vi "Dust_Control_Giraffe_small.vi"(7 "error in":errorcluster) -> (0 "error out":errorcluster)   [LabVIEW 2013]
doc: "This VI specifies the properties of the pulse used for running the dust source. When program is stopped, the voltage is incrementally reduced to zero to avoid quick drops."
uses:
  <vilib>/Utility/miscctls.llb/LVPointTypeDef.ctl
  Global Variables/Action Items.ctl
  <vilib>/Utility/error.llb/DialogType.ctl
  <vilib>/DAQmx/read.llb/DAQmx Read (Analog 1D Wfm NChan NSamp).vi
  <vilib>/Analysis/baseanly.llb/Mean (DBL).vi
  <vilib>/DAQmx/write.llb/DAQmx Write (Analog 1D Wfm NChan NSamp).vi
  <vilib>/DAQmx/read.llb/DAQmx Read (Counter U32 1Chan 1Samp).vi
  <vilib>/addons/database/Connection.llb/Conn Execute.vi
  <vilib>/addons/database/Recordset.llb/Rec Fetch Recordset Data (R).vi
  <vilib>/addons/database/Recordset.llb/Rec Destroy - Connection.vi
  <vilib>/DAQmx/create/channels.llb/DAQmx Create Channel (AI-Voltage-Basic).vi
  <vilib>/DAQmx/configure/timing.llb/DAQmx Timing (Sample Clock).vi
  <vilib>/DAQmx/create/channels.llb/DAQmx Create Channel (AO-Voltage-Basic).vi
  <vilib>/DAQmx/create/channels.llb/DAQmx Create Channel (CI-Count Edges).vi
  <userlib>/_OpenG.lib/comparison/comparison.llb/DBL Changed__ogtk.vi
  <vilib>/measure/mascope.llb/Amplitude and Levels 1 chan.vi
  <vilib>/DAQmx/miscellaneous.llb/DAQmx Fill In Error Info.vi
  Global Variables/throttle.vi
  <userlib>/_OpenG.lib/comparison/comparison.llb/Boolean Changed__ogtk.vi
  Global Variables/throttle from query.vi
  Sub-Polymorphic/post_dust_event_big.vi
  Sub-Polymorphic/post_dust_source_small.vi
  <vilib>/addons/database/_DB Variant To Data/Database Variant To Data.xnode
  <resource>/objmgr/daqmx.rc
  <vilib>/measure/NI_MAPro.lvlib
  <vilib>/Analysis/NI_AALBase.lvlib
  <vilib>/addons/database/NI_Database_API.lvlib
panel:
  out "Freq. Before Throttle":dbl
  out "On/Off":bool
  out "Finished":bool=TRUE
  out "Output waveform":waveform(dbl)={"t0"=timestamp(0 s since 1904-01-01), "dt"=4e-06, "Y"=array[50000 elements]}
  out "Input waveform":waveform(dbl)={"t0"=timestamp(3437998856.0330505 s since 1904-01-01), "dt"=0.00019999999999999998, "Y"=array[1000 elements], "attributes"=variant("NI_ChannelName"=variant(string "Dev5/ai20"), "NI_UnitDescription"=variant(string "Volts"))}
  out "output cluster":T1={"Integer Timestamp"=0, "Needle Voltage"=0.0, "Frequency"=1.0, "Width (ms) : 0.1 "=0.1, "Desired Amplitude (V)"=0.0, "Settings ID"="", "ID#"=0} {"Needle Voltage" min=0.0 max=10.0 step=0.01 format="%.2g"; "Desired Amplitude (V)" min=0.0 max=10.0 step=0.01 format="%5.2f"; "Width (ms) : 0.1" min=0.05 max=5.0 step=0.01 format="%6.2f"; "Frequency" min=1.0 max=100.0 step=0.01 format="%.1f"}
  in  "Tab Control":enum32{"Controls", "Status", "Counter"}(tab)
  in  "Big Accelerator\nSetting?":bool
  out "Actual output width (ms)":dbl caption="Actual Output Width (ms)" format="%.2f"
  out "Actual output Frequency":dbl caption="Actual Output  Frequency (hz)" format="%.2f"
  in  "Width (ms) : 0.1":dbl=0.1 min=0.0 max=5.0 step=0.01 format="%6.2f"
  out "Actual Amplitude (V) 2":dbl=0.0012999050305587314 caption="Actual Amplitude (V)" format="%.2f"
  in  "Desired Amplitude (V)":dbl min=0.0 max=10.0 step=0.01 format="%5.2f"
  out "Actual output Amplitude (V)":dbl caption="Actual Output Amplitude (V)" format="%.2f"
  in  "Frequency":dbl=1.0 caption="Frequency (Hz) : 1" min=0.0 max=30.0 step=0.01 format="%.1f"
  in  "Abort Change":bool
  out "Actual Needle (kV)":dbl=-1.1093266413053247 caption="Actual Einzel (V)" format="%.2f"
  out "Actual Needle Output (V)":dbl caption="Actual Einzel (V)" format="%.2f"
  in  "Needle Voltage":dbl min=0.0 max=10.0 step=0.01 format="%.2g"
  in  "Save Settings?":bool
  out "CONTROLS":waveform(dbl)[](graph)=[{"t0"=timestamp(0 s since 1904-01-01), "dt"=4e-06, "Y"=array[50000 elements]}, {"t0"=timestamp(3437998856.0330505 s since 1904-01-01), "dt"=0.00019999999999999998, "Y"=array[1000 elements], "attributes"=variant("NI_ChannelName"=variant(string "Dev5/ai20"), "NI_UnitDescription"=variant(string "Volts"))}]
  in  "Settings ID":string
  in  "Retrieve Settings":bool
  out "Ratio of particles at\nsecond detector to first":dbl
  out "First detector since\nlast source change:":i64
  out "Average Rate of first":dbl
  out "Average Rate of second":dbl
  in  "# of Cycles ot Average":i32=10
  out "Number of Hours":dbl
  out "Chamber Pressure":dbl format="%#_3g"
  in  "Physical Channels":tag="Dev4/ao0:1" caption="Physical Output Channels"
  in  "Physical Input Channels":tag="Dev6/ai0:2"
  out "Execution Number:":i32=341
  out "Testing":bool
  in  "Counters On/Off":bool=TRUE
  in  "Reset Counters":bool
  in  "Det1":tag="Dev5/ctr0"
  in  "Det2":tag="Dev5/ctr1"
  out "Det2":u32
  out "Det1":u32
  out "error?":bool
  out "Actual Sample Clock Rate":dbl=250000.0 format="%.2f"
  in  "stop":bool
  # "CCLDAS Dust Control Small Accelerator"
  # "Hold Down to\nStop Changes"
  # "Tube Drive (Ao0, Ai4)"
  # "Needle Control (Ao4, Ai0)"
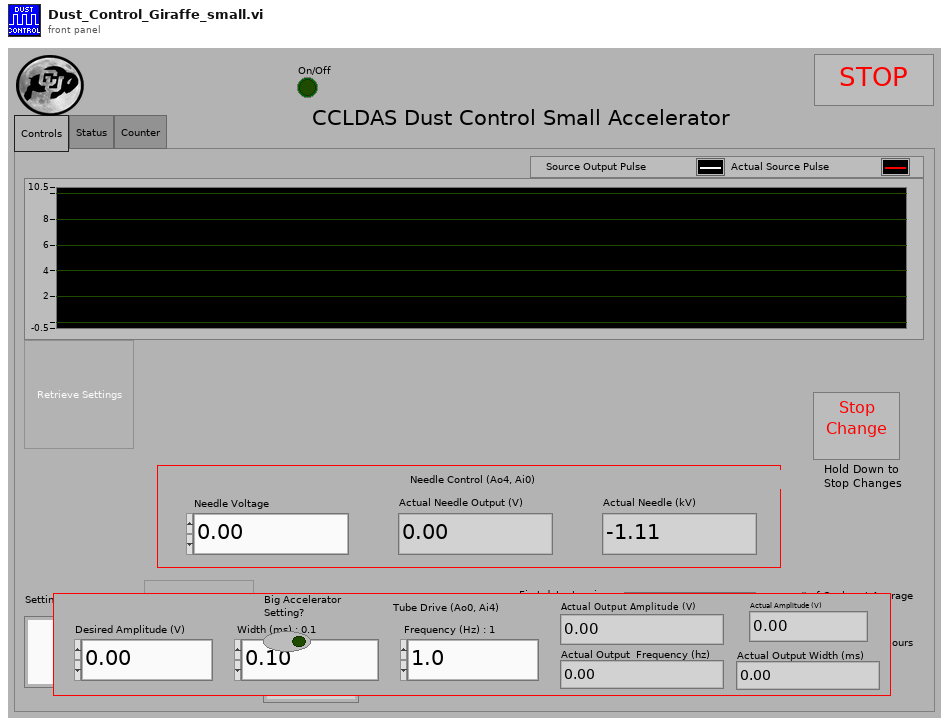
[diagram p1: front panel]
types:
  T1 = cluster{"Integer Timestamp":u64, "Needle Voltage":dbl, "Frequency":dbl, "Width (ms) : 0.1 ":dbl, "Desired Amplitude (V)":dbl, "Settings ID":string, "ID#":i32}
  T2 = typedef "Action Items.ctl" = enum16{"Initialize", "Get", "Set"}
  T3 = typedef "LVPointTypeDef.ctl" = cluster{"Horizontal":i16, "Vertical":i16}
  T4 = typedef "NI_Database_API.lvlib/Conn ObjectReference.ctl" = refnum<k1>
  T5 = typedef "NI_Database_API.lvlib/Rec ObjectReference.ctl" = refnum<k1>
  T6 = enum8{"Enabled", "Disabled", "Disabled and Grayed Out"}
  T7 = typedef "DialogType.ctl" = u16
  T8 = typedef "dust_source_control.ctl" = cluster{"Integer Timestamp":u64, "Einzel Voltage":dbl, "Needle Voltage":dbl, "Frequency":dbl, "Width (ms) : 0.1 ":dbl, "Desired Amplitude (V)":dbl, "X Voltage":dbl, "Y Voltage":dbl, "Settings ID":string, "ID#":i32}
  T9 = cluster{"Integer Time":i64, "Integer Time":i64, "data":i32}
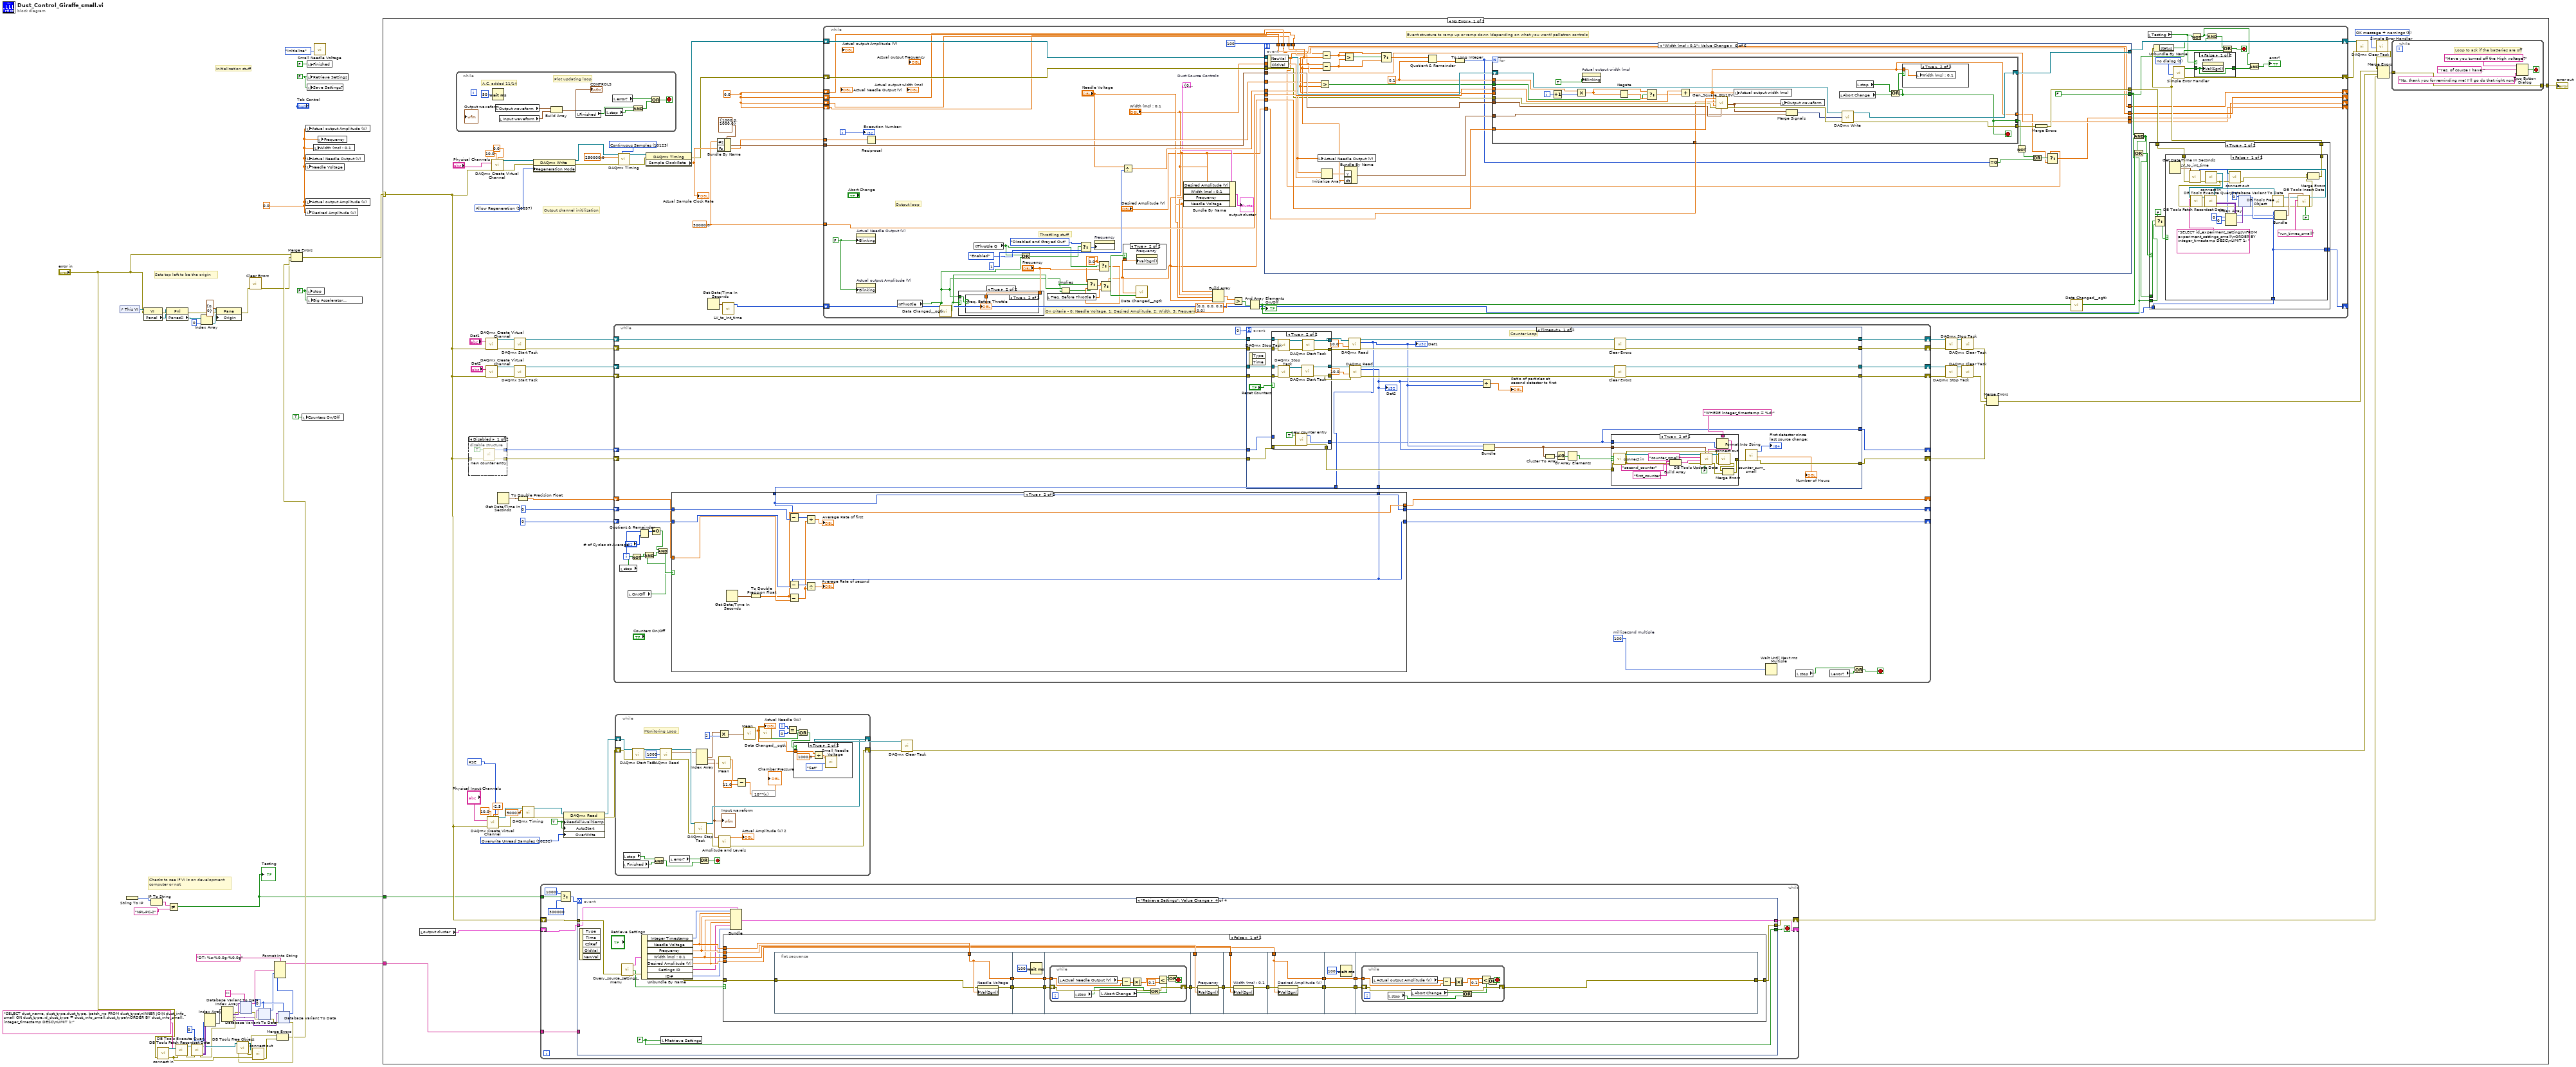
[diagram p0: block diagram]
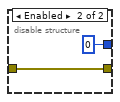
[diagram p2: hidden frame]
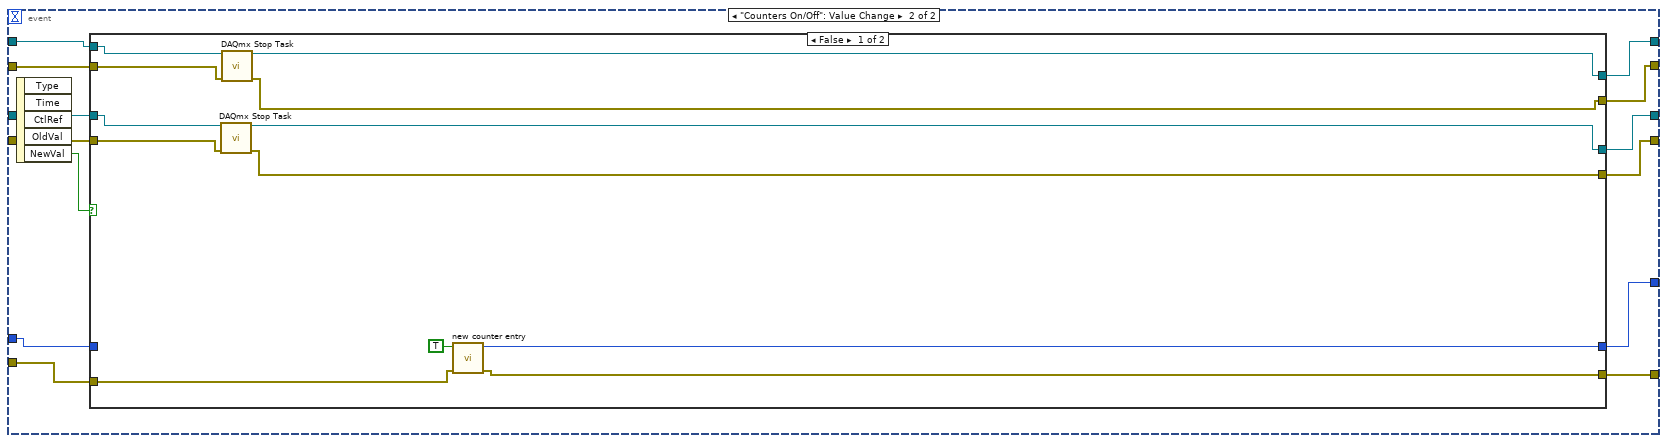
[diagram p5: hidden frame]
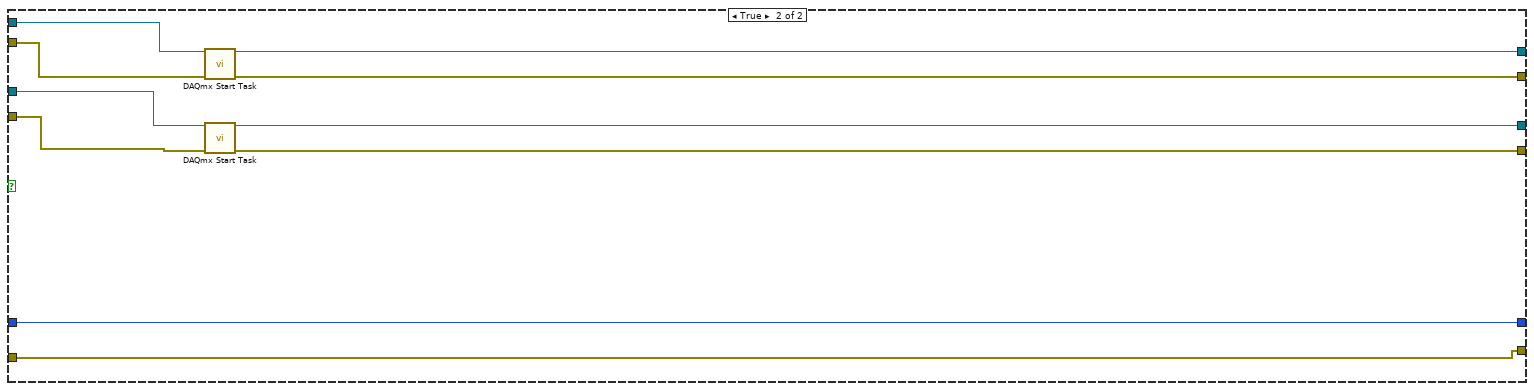
[diagram p6: hidden frame]
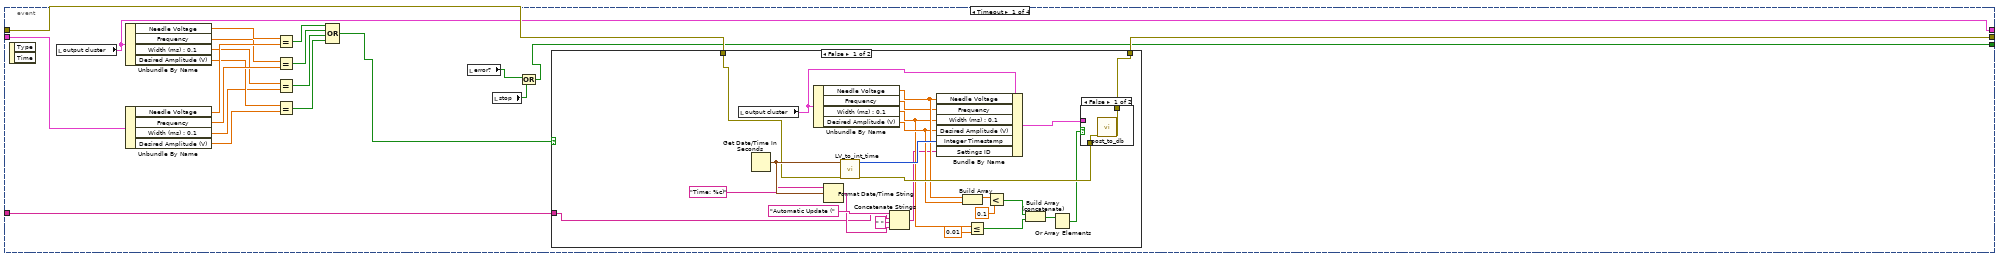
[diagram p9: hidden frame]
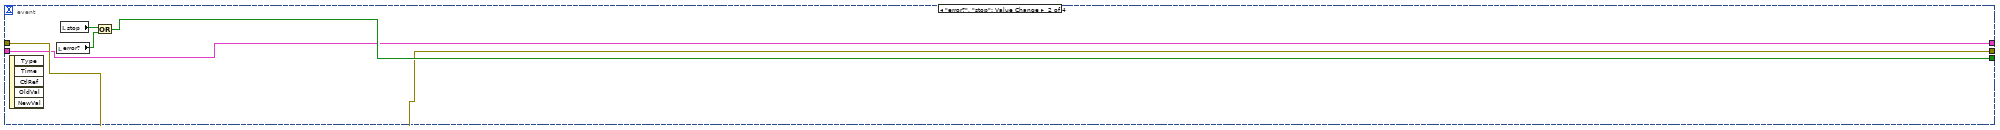
[diagram p12: hidden frame]
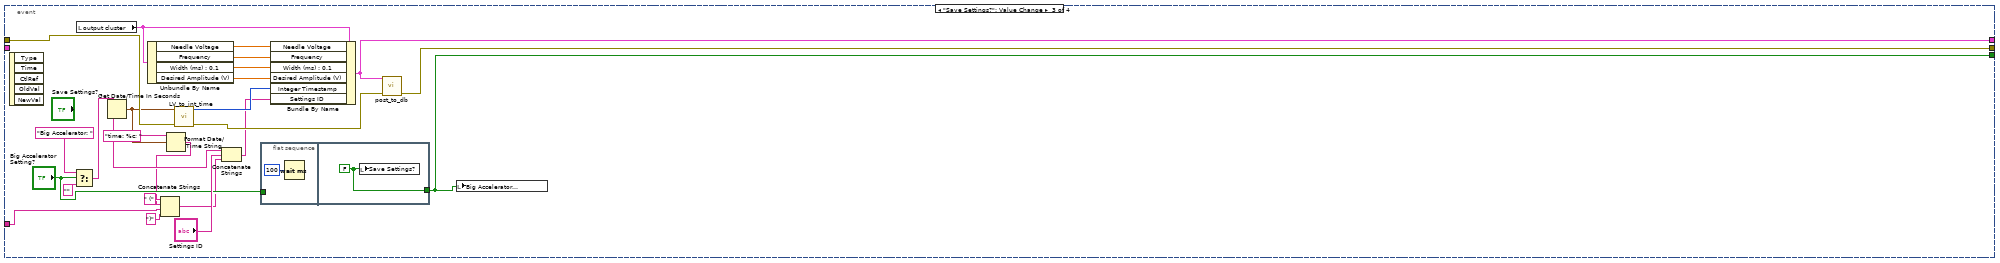
[diagram p13: hidden frame]
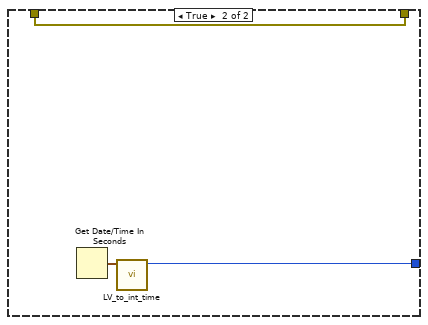
[diagram p19: hidden frame]
diagram:
  w13 = 0
  w48 = FALSE ("Retrieve Settings")
  w46 = 0.0 ("Actual Output (V)")
  w45 = FALSE ("Shutdown")
  # "Checks to see if VI is on development\ncomputer or not"
  # "Sets top left to be the origin"
  # "Initialization stuff"
  n1 = control-ref of="This VI"() -> (w44:refnum<vi>)
  n2 = String To IP() -> (0:w36:u32)  [unwired: 1 in]
  n3 = property class="VI"(reference=w44, error in="error in") -> (error out=w43:errorcluster, "Panel"=w42:refnum<vi>)  [unwired: 1 out]
  n4 = IP To String(2:w36) -> (0:w35:string)  [unwired: 1 in]
  n5 = call "connect in.vi"("error in (no error)"="error in") -> ("error out"=w30:errorcluster, "Database Connection"=w33:T4)  [unwired: 7 in]
  n6 = property class="Pnl"(reference=w42, error in=w43) -> (error out=w41:errorcluster, "Panes[]"=w40:refnum<vi>[])  [unwired: 1 out]
  n7 = Not Equal?(x=w35, y="NPL-PC-2") -> (x != y?=w6:bool)
  "Testing" <- w6
  n8 = call-poly <vilib>:"DB Tools Execute Query.vi"("error in (no error)"=w30, "SQL query"="SELECT dust_name, dust_type.dust_type, batch_no FROM dust_type\nINNER JOIN dust_info_small ON dust_type.id_dust_type = dust_info_small.dust_type\nORDER BY dust_info_small.integer_timestamp DESC\nLIMIT 1;", "connection reference"=w33) -> ("error out"=w32:errorcluster, "recordset reference"=w31:T5)  [unwired: 5 in]
  n9 = call-poly <vilib>:"DB Tools Fetch Recordset Data.vi"("error in (no error)"=w32, "recordset reference"=w31) -> ("error out"=w18:errorcluster, "recordset data"=w28:variant[][], "recordset reference out"=w27:T5)  [unwired: 3 in]
  n10 = Index Array(array=w40, index=0) -> (element=w38:refnum<vi>)
  n11 = Index Array(array=w28, index (row)=0) -> (element=w22:variant[])  [unwired: 1 in]
  n12 = property class="Pane"(reference=w38, error in=w41, "Origin"=T3 {"Horizontal"=0, "Vertical"=0}) -> (error out=w3:errorcluster)  [unwired: 1 out]
  n13 = Index Array(array=w22) -> (element #1=w21:variant, element #2=w16:variant, element #3=w15:variant)  [unwired: 3 in]
  n14 = xnode "Database Variant To Data"("database variant"=w21, "error in (no error)"=w18, "type"="") -> ("data"=w11:string, "error out"=w20:errorcluster)
  n15 = call <vilib>:"Clear Errors.vi"("error in (no error)"=w3) -> ("error out"=w4:errorcluster)  [unwired: 6 in]
  n16 = xnode "Database Variant To Data"("database variant"=w16, "error in (no error)"=w20, "type"=w13) -> ("data"=w10:i32, "error out"=w19:errorcluster)
  n17 = xnode "Database Variant To Data"("database variant"=w15, "error in (no error)"=w19, "type"=w13) -> ("data"=w9:i32, "error out"=w17:errorcluster)
  n18 = call-poly <vilib>:"DB Tools Free Object.vi"("error in (no error)"=w17, "recordset reference"=w27) -> ("error out"=w26:errorcluster, "connection reference"=w23:T4)  [unwired: 8 in]
  n19 = call "connect out.vi"("error in (no error)"=w30, "connection reference"=w23) -> ("error out"=w25:errorcluster)  [unwired: 9 in]
  n20 = Format Into String(format string="DT: %s-%0.0g-%0.0g", w11, w10, w9) -> (resulting string=w7:string)  [unwired: 2 in, 1 out]
  n21 = Merge Errors(w26, w25) -> (w8:errorcluster)
  n22 = Merge Errors("error in", w4, w8) -> (w5:errorcluster)
  n23 = local write "Counters On/Off"(TRUE ("Counters On/Off")) -> ()
  n24 = local write "Actual output Amplitude (V)"(w46) -> ()
  n25 = local write "Actual Needle Output (V)"(w46) -> ()
  n26 = local write "Needle Voltage"(w46) -> ()
  n27 = local write "Actual output Amplitude (V)"(w46) -> ()
  n28 = local write "Desired Amplitude (V)"(w46) -> ()
  n29 = local write "Finished"(FALSE ("Finished")) -> ()
  n30 = local write "Retrieve Settings"(w48) -> ()
  n31 = local write "Save Settings?"(w48) -> ()
  n32 = local write "stop"(w45) -> ()
  n33 = local write "Big Accelerator\nSetting?"(w45) -> ()
  n34 = local write "Width (ms) : 0.1"(w46) -> ()
  n35 = call "Small Needle Voltage.vi"("Action"=Action_Items."Initialize") -> ()  [unwired: 10 in, 1 out]
  n36 = local write "Frequency"(w46) -> ()
  n37 = case shown="No Error" w5 {
    selector: w5 -> [w63 w996]
    tunnel: [w105 w996] -> w50
    tunnel: w7 -> [w53 _]
    tunnel: w6 -> [w52 _]
    frame No Error {
      w51 = 10083 items=["default"=-1, "RSE"=10083, "NRSE"=10078, "Differential"=10106, "Pseudodifferential"=12529] ("input terminal configuration")
      w60 = 0.0 ("Width (ms) : 3.5")
      w73 = 10252 items=["Overwrite Unread Samples"=10252, "Do Not Overwrite Unread Samples"=10159] ("OverWrite")
      w74 = TRUE ("ReadAllAvailSamp")
      w56 = 50000.0 ("Size (Samples)")
      w118 = 10097 items=["Allow Regeneration"=10097, "Do Not Allow Regeneration"=10158] ("RegenMode")
      w123 = T7 3 items=["no dialog", "OK message", "continue or stop message", "OK message + warnings", "continue/stop + warnings"] ("type of dialog (OK msg:1)")
      w127 = 10123 items=["Finite Samples"=10178, "Continuous Samples"=10123] ("sample mode")
      # "Output channel initilization"
      n38 = local read "output cluster"() -> (w55:T1)
      n39 = while {
        stop <- w302 stop-if-true
        # "Plot updating loop"
        # "A.C. added 11/14"
        n40 = Wait (ms)(milliseconds to wait=u32 50) -> ()  [unwired: 1 out]
        n41 = local read "Output waveform"() -> (w299:waveform(dbl))
        n42 = local read "Input waveform"() -> (w300:waveform(dbl))
        n43 = Build Array(w299, w300) -> (→"CONTROLS":waveform(dbl)[])
        n44 = local read "Finished"() -> (w297:bool)
        n45 = local read "stop"() -> (w298:bool)
        n46 = local read "error?"() -> (w301:bool)
        n47 = And(x=w297, y=w298) -> (x .and. y?=w296:bool)
        n48 = Or(x=w301, y=w296) -> (x .or. y?=w302:bool)
      }
      n49 = disable-structure shown="Disabled" {
        disable-tunnel: [w131 w133] -> w82
        disable-tunnel: [w130 i64 0 ("Integer Time")] -> w81
        disable-tunnel: w63 -> [w129 w133]
        frame Disabled {
          n50 = call "new counter entry.vi"("error in"=w129, "Small?"=TRUE) -> ("error out"=w131:errorcluster, "Integer Time"=w130:i64)  [unwired: 8 in]
        }
        frame Enabled {
        }
      }
      n51 = call-poly <vilib>:"DAQmx Create Virtual Channel.vi"("counter"="Det1", "error in"=w63) -> ("task out"=w90:refnum<k21>, "error out"=w87:errorcluster)  [unwired: 12 in]
      n52 = call-poly <vilib>:"DAQmx Create Virtual Channel.vi"("counter"="Det2", "error in"=w63) -> ("task out"=w89:refnum<k21>, "error out"=w88:errorcluster)  [unwired: 12 in]
      n53 = call-poly <vilib>:"DAQmx Create Virtual Channel.vi"("maximum value"=10.0 ("Maximum Value"), "minimum value"=-2.5 ("Minimum Value"), "input terminal configuration"=w51, "physical channels"="Physical Input Channels", "error in"=w63) -> ("task out"=w67:refnum<k21>, "error out"=w66:errorcluster)  [unwired: 9 in]
      n54 = call-poly <vilib>:"DAQmx Create Virtual Channel.vi"("maximum value"=10.0 ("Maximum Value"), "minimum value"=0.0 ("Minimum Value"), "physical channels"="Physical Channels", "error in"=w63) -> ("task out"=w117:refnum<k21>, "error out"=w116:errorcluster)  [unwired: 10 in]
      n55 = Get Date/Time In Seconds() -> (seconds since 1Jan1904=w80:timestamp)
      n56 = call <vilib>:"DAQmx Start Task.vi"("task/channels in"=w90, "error in"=w87) -> ("task out"=w102:refnum<k21>, "error out"=w99:errorcluster)  [unwired: 12 in]
      n57 = call <vilib>:"DAQmx Start Task.vi"("task/channels in"=w89, "error in"=w88) -> ("task out"=w101:refnum<k21>, "error out"=w100:errorcluster)  [unwired: 12 in]
      n58 = To Double Precision Float(number=w80) -> (double precision float=w79:dbl)
      n59 = call-poly <vilib>:"DAQmx Timing.vi"("task/channels in"=w67, "rate"=5000.0, "error in"=w66) -> ("task out"=w72:refnum<k21>, "error out"=w71:errorcluster)  [unwired: 11 in]
      n60 = property class="DAQmx Write"(reference=w117, error in=w116, "Regeneration Mode"=w118) -> (reference out=w115:refnum<k21>, error out=w114:errorcluster)
      n61 = while {
        shift-right: [w348] -> w84
        shift-left: w63 -> [w347]
        shift-right: [w340] -> _
        shift-left: w55 -> [w349]
        tunnel: w52 -> [w343]
        tunnel: w53 -> [w341]
        stop <- w346 stop-if-true
        n62 = Select(t=1000, s=w343, f=300000) -> (s? t:f=w345:i32)
        n63 = event shown="[3] \"Retrieve Settings\": Value Change" {
          selector: _ -> [_ _ _ _]
          dyn-events: _ -> [_ _ _ _]
          timeout: w345 -> [_ _ _ _]
          tunnel: [w350 w399 w404 w430] -> w340
          tunnel: w349 -> [w370 w399 _ w438]
          tunnel: [w355 w400 w427 w444] -> w348
          tunnel: w347 -> [w356 w400 w424 w442]
          tunnel: [w353 w401 w413 w443] -> w346
          tunnel: w341 -> [w357 _ w410 _]
          event Timeout {
            n64 = event-data() -> ()  [unwired: 1 in, 2 out]
            n65 = local read "output cluster"() -> (w350:T1)
            n66 = Unbundle By Name(w350) -> ("Needle Voltage"=w369:dbl, "Frequency"=w367:dbl, "Width (ms) : 0.1"=w365:dbl, "Desired Amplitude (V)"=w363:dbl)
            n67 = Unbundle By Name(w370) -> ("Needle Voltage"=w368:dbl, "Frequency"=w366:dbl, "Width (ms) : 0.1"=w358:dbl, "Desired Amplitude (V)"=w364:dbl)
            n68 = Equal?(x=w369, y=w368) -> (x = y?=w362:bool)
            n69 = Equal?(x=w367, y=w366) -> (x = y?=w361:bool)
            n70 = Equal?(x=w365, y=w358) -> (x = y?=w360:bool)
            n71 = Equal?(x=w363, y=w364) -> (x = y?=w359:bool)
            n72 = Compound Arithmetic op=OR(w362, w361, w360, w359) -> (w354:bool)
            n73 = local read "error?"() -> (w352:bool)
            n74 = local read "stop"() -> (w351:bool)
            n75 = Or(x=w352, y=w351) -> (x .or. y?=w353:bool)
            n76 = case shown="False" w354 {
              tunnel: w357 -> [w371 _]
              tunnel: w356 -> [w376 w398]
              tunnel: [w375 w398] -> w355
              frame False {
                n77 = local read "output cluster"() -> (w380:T1)
                n78 = Get Date/Time In Seconds() -> (seconds since 1Jan1904=w392:timestamp)
                n79 = Unbundle By Name(w380) -> ("Needle Voltage"=w390:dbl, "Frequency"=w386:dbl, "Width (ms) : 0.1"=w385:dbl, "Desired Amplitude (V)"=w389:dbl)
                n80 = Format Date/Time String(time format string (%c)="Time: %c)" ("Settings ID"), seconds (now)=w392) -> (date/time string=w372:string)  [unwired: 1 in]
                n81 = call "LV_to_int_time.vi"("error in (no error)"=w376, "Time Stamp"=w392) -> ("error out"=w393:errorcluster, "Integer Time"=w394:i64)  [unwired: 7 in]
                n82 = Concatenate Strings("Automatic Update (" ("string"), w371, " " ("string"), w372) -> (w378:string)
                n83 = Bundle By Name(cluster=w380, "Needle Voltage"=w390, "Frequency"=w386, "Width (ms) : 0.1"=w385, "Desired Amplitude (V)"=w389, "Integer Timestamp"=w394, "Settings ID"=w378) -> (w381:T1)
                n84 = Build Array(w390, w389) -> (w388:dbl[])
                n85 = Less Or Equal?(x=w385, y=0.01) -> (x <= y?=w379:bool)
                n86 = Less?(x=w388, y=0.1) -> (x < y?=w383:bool[])
                n87 = Build Array (concatenate)(w383, w379) -> (w382:bool[])
                n88 = Or Array Elements(Boolean array=w382) -> (logical OR=w377:bool)
                n89 = case shown="False" w377 {
                  tunnel: w381 -> [_ _]
                  tunnel: [w396 w397] -> w375
                  tunnel: w393 -> [w395 w397]
                  frame False {
                    n90 = call-poly "post_to_db.vi"("error in (no error)"=w395) -> ("error out"=w396:errorcluster)  [unwired: 8 in, 2 out]
                  }
                  frame True {
                  }
                }
              }
              frame True {
              }
            }
          }
          event "error?", "stop": Value Change {
            n91 = event-data() -> ()  [unwired: 1 in, 5 out]
            n92 = local read "error?"() -> (w402:bool)
            n93 = local read "stop"() -> (w403:bool)
            n94 = Or(x=w403, y=w402) -> (x .or. y?=w401:bool)
          }
          event "Save Settings?": Value Change {
            n95 = event-data() -> ()  [unwired: 1 in, 5 out]
            n96 = Select(t="Big Accelerator: ", s="Big Accelerator\nSetting?", f="") -> (s? t:f=w415:string)
            n97 = local read "output cluster"() -> (w405:T1)
            n98 = Get Date/Time In Seconds() -> (seconds since 1Jan1904=w422:timestamp)
            n99 = Unbundle By Name(w405) -> ("Needle Voltage"=w421:dbl, "Frequency"=w420:dbl, "Width (ms) : 0.1"=w419:dbl, "Desired Amplitude (V)"=w418:dbl)
            n100 = Format Date/Time String(time format string (%c)="time: %c; " ("Settings ID"), seconds (now)=w422) -> (date/time string=w408:string)  [unwired: 1 in]
            n101 = Concatenate Strings(" (" ("string"), w408, w410, ")" ("string")) -> (w407:string)
            n102 = call "LV_to_int_time.vi"("error in (no error)"=w424, "Time Stamp"=w422) -> ("error out"=w425:errorcluster, "Integer Time"=w426:i64)  [unwired: 7 in]
            n103 = Concatenate Strings(w415, "Settings ID", w407) -> (w406:string)
            n104 = flat-sequence {
              tunnel: "Big Accelerator\nSetting?" -> [_]
              tunnel: [w429] -> w413
              frame #0 {
                n105 = Wait (ms)(milliseconds to wait=u32 100) -> ()  [unwired: 1 out]
              }
              frame #1 {
                w429 = FALSE
                n106 = local write "Save Settings?"(w429) -> ()
              }
            }
            n107 = Bundle By Name(cluster=w405, "Needle Voltage"=w421, "Frequency"=w420, "Width (ms) : 0.1"=w419, "Desired Amplitude (V)"=w418, "Integer Timestamp"=w426, "Settings ID"=w406) -> (w404:T1)
            n108 = call-poly "post_to_db.vi"("error in (no error)"=w425, "Dust control settings"=w404) -> ("error out"=w427:errorcluster)  [unwired: 9 in]
            n109 = local write "Big Accelerator\nSetting?"(w413) -> ()
          }
          event "Retrieve Settings": Value Change {
            w443 = FALSE
            n110 = event-data() -> ()  [unwired: 1 in, 5 out]
            n111 = call "Query_source_settings_menu.vi"("error in (no error)"=w442) -> ("error out"=w440:errorcluster, "Cancelled?"=w439:bool, "Output cluster"=w441:T8)  [unwired: 8 in]
            n112 = Unbundle By Name(w441) -> ("Integer Timestamp"=w433:u64, "Needle Voltage"=w437:dbl, "Frequency"=w436:dbl, "Width (ms) : 0.1"=w435:dbl, "Desired Amplitude (V)"=w434:dbl, "Settings ID"=w432:string, "ID#"=w431:i32)
            n113 = local write "Retrieve Settings"(w443) -> ()
            n114 = case shown="False" w439 {
              tunnel: w440 -> [w461 w508]
              tunnel: w437 -> [w460 _]
              tunnel: w436 -> [w459 _]
              tunnel: w435 -> [w457 _]
              tunnel: w434 -> [w448 _]
              tunnel: [w445 w508] -> w444
              frame False {
                n115 = flat-sequence {
                  tunnel: w460 -> [w463]
                  tunnel: [w464] -> w456
                  tunnel: [w463] -> w452
                  tunnel: w461 -> [w462]
                  tunnel: w456 -> [w467]
                  tunnel: [w467] -> w455
                  tunnel: [w465] -> w453
                  tunnel: w452 -> [w465]
                  tunnel: w455 -> [w469]
                  tunnel: w453 -> [w470]
                  tunnel: [w468] -> w451
                  tunnel: w459 -> [w484]
                  tunnel: [w483] -> w458
                  tunnel: w451 -> [w482]
                  tunnel: w458 -> [w487]
                  tunnel: w457 -> [w485]
                  tunnel: [w486] -> w450
                  tunnel: w450 -> [w490]
                  tunnel: [w488] -> w449
                  tunnel: w448 -> [w489]
                  tunnel: [w489] -> w447
                  tunnel: w449 -> [w493]
                  tunnel: [w493] -> w454
                  tunnel: w447 -> [w491]
                  tunnel: [w491] -> w446
                  tunnel: [w496] -> w445
                  tunnel: w454 -> [w495]
                  tunnel: w446 -> [w494]
                  frame #0 {
                    n116 = property on="Needle Voltage" class="DigNum (strict)"(error in=w462, "Val(Sgnl)"=w463) -> (error out=w464:errorcluster)  [unwired: 1 in, 1 out]
                  }
                  frame #1 {
                    n117 = Wait (ms)(milliseconds to wait=u32 100) -> ()  [unwired: 1 out]
                  }
                  frame #2 {
                    n118 = while {
                      tunnel: w470 -> [w476]
                      shift-right: [w481] -> w468
                      shift-left: w469 -> [w481]
                      stop <- w474 stop-if-true
                      n119 = local read "Actual Needle Output (V)"() -> (w477:dbl)
                      n120 = local read "stop"() -> (w471:bool)
                      n121 = local read "Abort Change"() -> (w473:bool)
                      n122 = Subtract(x=w477, y=w476) -> (x-y=w480:dbl)
                      n123 = Absolute Value(x=w480) -> (abs(x)=w479:dbl)
                      n124 = Or(x=w471, y=w473) -> (x .or. y?=w472:bool)
                      n125 = Less?(x=w479, y=0.1) -> (x < y?=w475:bool)
                      n126 = Or(x=w472, y=w475) -> (x .or. y?=w474:bool)
                    }
                  }
                  frame #3 {
                    n127 = property on="Frequency" class="DigNum (strict)"(error in=w482, "Val(Sgnl)"=w484) -> (error out=w483:errorcluster)  [unwired: 1 in, 1 out]
                  }
                  frame #4 {
                    n128 = property on="Width (ms) : 0.1" class="DigNum (strict)"(error in=w487, "Val(Sgnl)"=w485) -> (error out=w486:errorcluster)  [unwired: 1 in, 1 out]
                  }
                  frame #5 {
                    n129 = property on="Desired Amplitude (V)" class="DigNum (strict)"(error in=w490, "Val(Sgnl)"=w489) -> (error out=w488:errorcluster)  [unwired: 1 in, 1 out]
                  }
                  frame #6 {
                    n130 = Wait (ms)(milliseconds to wait=u32 100) -> ()  [unwired: 1 out]
                  }
                  frame #7 {
                    n131 = while {
                      tunnel: w494 -> [w507]
                      shift-right: [w505] -> w496
                      shift-left: w495 -> [w505]
                      stop <- w500 stop-if-true
                      n132 = local read "Actual output Amplitude (V)"() -> (w506:dbl)
                      n133 = local read "stop"() -> (w497:bool)
                      n134 = local read "Abort Change"() -> (w498:bool)
                      n135 = Subtract(x=w506, y=w507) -> (x-y=w503:dbl)
                      n136 = Absolute Value(x=w503) -> (abs(x)=w502:dbl)
                      n137 = Or(x=w498, y=w497) -> (x .or. y?=w499:bool)
                      n138 = Less?(x=w502, y=0.1) -> (x < y?=w504:bool)
                      n139 = Or(x=w504, y=w499) -> (x .or. y?=w500:bool)
                    }
                  }
                }
              }
              frame True {
              }
            }
            n140 = Bundle(cluster=w438, "Integer Timestamp"=w433, "Needle Voltage"=w437, "Frequency"=w436, "Width (ms) : 0.1"=w435, "Desired Amplitude (V)"=w434, "Settings ID"=w432, "ID#"=w431) -> (w430:T1)
          }
        }
      }
      n141 = property class="DAQmx Read"(reference=w72, error in=w71, "ReadAllAvailSamp"=w74, "AutoStart"=w74, "OverWrite"=w73) -> (reference out=w64:refnum<k21>, error out=w62:errorcluster)
      n142 = while {
        shift-right: [w153] -> _
        shift-left: w81 -> [w155]
        shift-right: [w148] -> _
        shift-left: w79 -> [w144]
        shift-right: [w147] -> _
        shift-left: u32 0 ("data") -> [w151]
        shift-right: [w146] -> _
        shift-left: u32 0 ("data") -> [w150]
        shift-right: [w167] -> w98
        shift-left: w102 -> [w159]
        shift-right: [w161] -> w97
        shift-left: w99 -> [w158]
        shift-right: [w166] -> w96
        shift-left: w101 -> [w157]
        shift-right: [w165] -> w95
        shift-left: w100 -> [w156]
        shift-right: [w160] -> w57
        shift-left: w82 -> [w154]
        i -> [w136]
        stop <- w162 stop-if-true
        w164 = u32 100  # millisecond multiple
        n143 = local read "stop"() -> (w143:bool)
        n144 = local read "On/Off"() -> (w135:bool)
        n145 = Not(x=w143) -> (.not. x?=w142:bool)
        n146 = Quotient & Remainder(x=w136, y="# of Cycles ot Average") -> (x-y*floor(x/y)=w145:i32)  [unwired: 1 out]
        n147 = And(x=w142, y=w135) -> (x .and. y?=w139:bool)
        n148 = Equal To 0?(x=w145) -> (x = 0?=w140:bool)
        n149 = And(x=w140, y=w139) -> (x .and. y?=w141:bool)
        n150 = event shown="[0] Timeout" {
          selector: _ -> [_ _]
          dyn-events: _ -> [_ _]
          timeout: 0 -> [_ _]
          tunnel: [w200 w249] -> w167
          tunnel: [w197 w247] -> w166
          tunnel: [w196 w246] -> w165
          tunnel: [w192 w248] -> w161
          tunnel: [w191 w240] -> w160
          tunnel: w159 -> [w188 w244]
          tunnel: w158 -> [w187 w251]
          tunnel: w157 -> [w186 w245]
          tunnel: w156 -> [w185 w250]
          tunnel: w155 -> [w179 w243]
          tunnel: w154 -> [w178 w241]
          tunnel: [w169 w242] -> w153
          tunnel: [w175 _] -> w149
          tunnel: [w170 _] -> w134
          event Timeout {
            # "Counter Loop"
            n151 = event-data() -> ()  [unwired: 1 in, 2 out]
            n152 = case shown="True" "Reset Counters" {
              tunnel: w188 -> [w223 w239]
              tunnel: [w223 w237] -> w184
              tunnel: w187 -> [w222 w236]
              tunnel: [w222 w234] -> w183
              tunnel: w186 -> [w221 w233]
              tunnel: [w221 w231] -> w182
              tunnel: w185 -> [w220 w230]
              tunnel: [w220 w228] -> w181
              tunnel: w178 -> [w219 w226]
              tunnel: [w218 w227] -> w169
              tunnel: [w219 w225] -> w177
              tunnel: w179 -> [w218 _]
              frame False {
              }
              frame True {
                n153 = call <vilib>:"DAQmx Stop Task.vi"("task/channels in"=w233, "error in"=w230) -> ("task out"=w232:refnum<k21>, "error out"=w229:errorcluster)  [unwired: 12 in]
                n154 = call <vilib>:"DAQmx Stop Task.vi"("task/channels in"=w239, "error in"=w236) -> ("task out"=w238:refnum<k21>, "error out"=w235:errorcluster)  [unwired: 12 in]
                n155 = call "new counter entry.vi"("error in"=w226, "Small?"=TRUE) -> ("error out"=w225:errorcluster, "Integer Time"=w227:i64)  [unwired: 8 in]
                n156 = call <vilib>:"DAQmx Start Task.vi"("task/channels in"=w232, "error in"=w229) -> ("task out"=w231:refnum<k21>, "error out"=w228:errorcluster)  [unwired: 12 in]
                n157 = call <vilib>:"DAQmx Start Task.vi"("task/channels in"=w238, "error in"=w235) -> ("task out"=w237:refnum<k21>, "error out"=w234:errorcluster)  [unwired: 12 in]
              }
            }
            n158 = call-poly <vilib>:"DAQmx Read.vi"("task/channels in"=w184, "timeout"=10.0, "error in"=w183) -> ("task out"=w200:refnum<k21>, "data"=w175:u32, "error out"=w195:errorcluster)  [unwired: 10 in]
            "Det1" <- w175
            n159 = call-poly <vilib>:"DAQmx Read.vi"("task/channels in"=w182, "timeout"=10.0, "error in"=w181) -> ("task out"=w197:refnum<k21>, "data"=w170:u32, "error out"=w194:errorcluster)  [unwired: 10 in]
            "Det2" <- w170
            n160 = Divide(x=w170, y=w175) -> (x/y=→"Ratio of particles at\nsecond detector to first":dbl)
            n161 = Bundle("data"=w175, "data"=w170) -> (w168:cluster{"data":u32, "data":u32})  [unwired: 1 in]
            n162 = Cluster To Array(cluster=w168) -> (array=w174:u32[])
            n163 = Not Equal To 0?(x=w174) -> (x != 0?=w173:bool[])
            n164 = Or Array Elements(Boolean array=w173) -> (logical OR=w172:bool)
            n165 = case shown="True" w172 {
              tunnel: [w201 w207] -> w190
              tunnel: "WHERE integer_timestamp = %d;" ("condition") -> [_ w206]
              tunnel: w177 -> [w201 w204]
              tunnel: w169 -> [_ w203]
              tunnel: w168 -> [_ w202]
              frame False {
              }
              frame True {
                n166 = call "connect in.vi"("error in (no error)"=w204) -> ("error out"=w210:errorcluster, "Database Connection"=w216:T4)  [unwired: 7 in]
                n167 = Build Array("first_counter" ("string"), "second_counter" ("string")) -> (w212:string[])
                n168 = Format Into String(format string=w206, w203) -> (resulting string=w205:string)  [unwired: 2 in, 1 out]
                n169 = call <vilib>:"DB Tools Update Data.vi"("condition"=w205, "flatten cluster? (F)"=FALSE ("create table? (F)"), "data"=w202, "error in (no error)"=w210, "columns"=w212, "table"="counter_small", "connection reference"=w216) -> ("error out"=w208:errorcluster, "connection reference out"=w214:T4)  [unwired: 3 in]
                n170 = call "connect out.vi"("error in (no error)"=w210, "connection reference"=w214) -> ("error out"=w209:errorcluster)  [unwired: 9 in]
                n171 = Merge Errors(w209, w208) -> (w207:errorcluster)
              }
            }
            n172 = call <vilib>:"Clear Errors.vi"("error in (no error)"=w195) -> ("error out"=w192:errorcluster)  [unwired: 6 in]
            n173 = call <vilib>:"Clear Errors.vi"("error in (no error)"=w194) -> ("error out"=w196:errorcluster)  [unwired: 6 in]
            n174 = call "counter_sum_small.vi"("error in"=w190) -> ("error IO"=w191:errorcluster, "Number of Hours"=→"Number of Hours":dbl, "First Detector Sum"=→"First detector since\nlast source change:":i64)  [unwired: 7 in, 1 out]
          }
          event "Counters On/Off": Value Change {
            n175 = event-data() -> ("NewVal"=w252:bool)  [unwired: 1 in, 4 out]
            n176 = case shown="False" w252 {
              tunnel: w251 -> [w263 w270]
              tunnel: w250 -> [w261 w269]
              tunnel: [w257 w274] -> w249
              tunnel: [w258 w273] -> w248
              tunnel: [w259 w272] -> w247
              tunnel: [w260 w271] -> w246
              tunnel: w245 -> [w262 w268]
              tunnel: w244 -> [w264 w267]
              tunnel: w243 -> [_ w266]
              tunnel: [w256 w266] -> w242
              tunnel: w241 -> [w255 w265]
              tunnel: [w254 w265] -> w240
              frame False {
                n177 = call <vilib>:"DAQmx Stop Task.vi"("task/channels in"=w262, "error in"=w261) -> ("task out"=w259:refnum<k21>, "error out"=w260:errorcluster)  [unwired: 12 in]
                n178 = call <vilib>:"DAQmx Stop Task.vi"("task/channels in"=w264, "error in"=w263) -> ("task out"=w257:refnum<k21>, "error out"=w258:errorcluster)  [unwired: 12 in]
                n179 = call "new counter entry.vi"("error in"=w255, "Small?"=TRUE) -> ("error out"=w254:errorcluster, "Integer Time"=w256:i64)  [unwired: 8 in]
              }
              frame True {
                n180 = call <vilib>:"DAQmx Start Task.vi"("task/channels in"=w267, "error in"=w270) -> ("task out"=w274:refnum<k21>, "error out"=w273:errorcluster)  [unwired: 12 in]
                n181 = call <vilib>:"DAQmx Start Task.vi"("task/channels in"=w268, "error in"=w269) -> ("task out"=w272:refnum<k21>, "error out"=w271:errorcluster)  [unwired: 12 in]
              }
            }
          }
        }
        n182 = case shown="True" w141 {
          tunnel: w144 -> [w277 w288]
          tunnel: w151 -> [w276 w287]
          tunnel: w150 -> [w275 w286]
          tunnel: w149 -> [_ w281]
          tunnel: [w277 w282] -> w148
          tunnel: [w276 w281] -> w147
          tunnel: [w275 w278] -> w146
          tunnel: w134 -> [_ w278]
          frame False {
          }
          frame True {
            n183 = Get Date/Time In Seconds() -> (seconds since 1Jan1904=w289:timestamp)
            n184 = To Double Precision Float(number=w289) -> (double precision float=w282:dbl)
            n185 = Subtract(x=w281, y=w287) -> (x-y=w285:u32)
            n186 = Subtract(x=w278, y=w286) -> (x-y=w284:u32)
            n187 = Subtract(x=w282, y=w288) -> (x-y=w283:dbl)
            n188 = Divide(x=w285, y=w283) -> (x/y=→"Average Rate of first":dbl)
            n189 = Divide(x=w284, y=w283) -> (x/y=→"Average Rate of second":dbl)
          }
        }
        n190 = Wait Until Next ms Multiple(millisecond multiple=w164) -> ()  [unwired: 1 out]
        n191 = local read "stop"() -> (w137:bool)
        n192 = local read "error?"() -> (w163:bool)
        n193 = Or(x=w137, y=w163) -> (x .or. y?=w162:bool)
      }
      n194 = while {
        shift-right: [w316] -> w61
        shift-left: w64 -> [w318]
        shift-right: [w319] -> w76
        shift-left: w62 -> [w317]
        i -> [w306]
        stop <- w320 stop-if-true
        # "Monitoring Loop"
        n195 = local read "stop"() -> (w334:bool)
        n196 = local read "Finished"() -> (w335:bool)
        n197 = call <vilib>:"DAQmx Start Task.vi"("task/channels in"=w318, "error in"=w317) -> ("task out"=w325:refnum<k21>, "error out"=w326:errorcluster)  [unwired: 12 in]
        n198 = And(x=w334, y=w335) -> (x .and. y?=w333:bool)
        n199 = call-poly <vilib>:"DAQmx Read.vi"("task/channels in"=w325, "number of samples per channel"=1000, "error in"=w326) -> ("task out"=w327:refnum<k21>, "data"=w321:waveform(dbl)[], "error out"=w328:errorcluster)  [unwired: 10 in]
        n200 = local read "error?"() -> (w322:bool)
        n201 = call <vilib>:"DAQmx Stop Task.vi"("task/channels in"=w327, "error in"=w328) -> ("task out"=w316:refnum<k21>, "error out"=w332:errorcluster)  [unwired: 12 in]
        n202 = Index Array(array=w321) -> (element #1=w323:waveform(dbl), element #2=w315:waveform(dbl), element #3=w314:waveform(dbl))  [unwired: 3 in]
        "Input waveform" <- w315
        n203 = Or(x=w322, y=w333) -> (x .or. y?=w320:bool)
        n204 = Multiply(x=w323, y=2) -> (x*y=w329:waveform(dbl))
        n205 = call-poly <vilib>:"Mean.vi"("X"=w314) -> ("mean"=w313:dbl)  [unwired: 1 out]
        n206 = call-poly <vilib>:"Amplitude and Levels.vi"("error in (no error)"=w332, "signal in"=w315) -> ("error out"=w319:errorcluster, "amplitude"=→"Actual Amplitude (V) 2":dbl)  [unwired: 6 in, 2 out]
        n207 = Subtract(x=w313, y=11.0) -> (x-y=w311:dbl)
        n208 = call-poly <vilib>:"Mean.vi"("X"=w329) -> ("mean"=w309:dbl)  [unwired: 1 out]
        "Actual Needle (kV)" <- w309
        n209 = expression code="10**(x)"(w311) -> (→"Chamber Pressure":dbl)
        n210 = call-poly <userlib>:"Data Changed__ogtk.vi"("DBL"=w309) -> ("Changed"=w307:bool)
        n211 = Equal?(x=w306, y=0) -> (x = y?=w304:bool)
        n212 = Or(x=w304, y=w307) -> (x .or. y?=w308:bool)
        n213 = case shown="True" w308 {
          tunnel: w309 -> [_ w337]
          frame False {
          }
          frame True {
            n214 = Divide(x=w337, y=1000.0) -> (x/y=w338:dbl)
            n215 = call "Small Needle Voltage.vi"("Action"=Action_Items."Set", "Input Pelletron Voltage"=w338) -> ()  [unwired: 9 in, 1 out]
          }
        }
      }
      n216 = call-poly <vilib>:"DAQmx Timing.vi"("task/channels in"=w115, "sample mode"=w127, "rate"=250000.0 ("Sample Clock Rate"), "error in"=w114) -> ("task out"=w121:refnum<k21>, "error out"=w107:errorcluster)  [unwired: 10 in]
      n217 = property class="DAQmx Timing"(reference=w121, error in=w107) -> (reference out=w109:refnum<k21>, error out=w54:errorcluster, "Sample Clock:Rate"=w113:dbl)
      "Actual Sample Clock Rate" <- w113
      n218 = Get Date/Time In Seconds() -> (seconds since 1Jan1904=w59:timestamp)
      n219 = Bundle By Name(cluster=cluster{"Fs":dbl, "#s":dbl} {"Fs"=1000.0, "#s"=1000.0} ("sampling info"), "#s"=w56, "Fs"=w113) -> (w119:cluster{"Fs":dbl, "#s":dbl})
      n220 = call "LV_to_int_time.vi"("Time Stamp"=w59) -> ("Integer Time"=w58:i64)  [unwired: 8 in, 1 out]
      n221 = while {
        tunnel: w119 -> [w568]
        tunnel: w113 -> [w566]
        tunnel: w56 -> [w555]
        shift-right: [w565] -> w112
        shift-left: w109 -> [w563]
        shift-right: [w562] -> w108
        shift-left: w54 -> [w570]
        shift-right: [w524] -> _
        shift-left: w60 -> [w528]
        shift-right: [w523] -> _
        shift-left: w60 -> [w527]
        shift-right: [w522] -> _
        shift-left: w60 -> [w526]
        shift-right: [w521] -> _
        shift-left: w60 -> [w525]
        shift-right: [w517] -> _
        shift-left: w58 -> [w518]
        i -> [w569]
        stop <- w511 stop-if-true
        w549 = 0.0 ("t")
        w557 = T1 {"Integer Timestamp"=0, "Needle Voltage"=1.0, "Frequency"=0.0, "Width (ms) : 0.1 "=0.0, "Desired Amplitude (V)"=0.0, "Settings ID"="", "ID#"=0}  # Dust Source Controls
        w561 = T7 0 items=["no dialog", "OK message", "continue or stop message", "OK message + warnings", "continue/stop + warnings"] ("type of dialog (OK msg:1)")
        w560 = FALSE ("Blinking")
        # "On criteria - 0: Needle Voltage, 1: Desired Amplitude, 2: Width, 3: Frequency"
        # "Event structure to ramp up or ramp down (depending on what you want) pelletron controls"
        # "Throttling stuff"
        # "Output loop"
        n222 = property on="Actual Needle Output (V)" class="DigNum (strict)"("Blinking"=w560) -> ()  [unwired: 2 in, 2 out]
        n223 = property on="Actual output Amplitude (V)" class="DigNum (strict)"("Blinking"=w560) -> ()  [unwired: 2 in, 2 out]
        n224 = Reciprocal(x=w566) -> (1/x=w567:dbl)
        n225 = global read "throttle.vi" "Throttle"() -> (w529:bool)
        n226 = call-poly <userlib>:"Data Changed__ogtk.vi"("Boolean"=w529) -> ("Changed"=w531:bool)
        n227 = case shown="True" w531 {
          tunnel: w529 -> [_ w574]
          tunnel: "Frequency" -> [_ w573]
          frame False {
          }
          frame True {
            n228 = case shown="True" w574 {
              tunnel: w573 -> [_ w575]
              frame False {
              }
              frame True {
                "Freq. Before Throttle" <- w575
              }
            }
          }
        }
        n229 = global read "throttle from query.vi" "Throttle Q"() -> (w550:bool)
        n230 = Or(x=w550, y=w529) -> (x .or. y?=w551:bool)
        n231 = local read "Freq. Before Throttle"() -> (w532:dbl)
        n232 = Implies(1:w529, 2:w531) -> (0:w530:bool)
        n233 = Select(t=T6."Disabled and Grayed Out" ("Disabled"), s=w551, f=T6."Enabled" ("Disabled")) -> (s? t:f=w552:T6)
        n234 = property on="Frequency" class="DigNum (strict)"("DisabledEnum"=w552) -> ()  [unwired: 2 in, 2 out]
        n235 = Select(t=w549, s=w550, f="Frequency") -> (s? t:f=w547:dbl)
        n236 = Select(t=w549, s=w529, f=w547) -> (s? t:f=w543:dbl)
        n237 = Select(t=w543, s=w530, f=w532) -> (s? t:f=w533:dbl)
        n238 = Divide(x="Needle Voltage", y=1) -> (x/y=w559:dbl)
        n239 = call-poly <userlib>:"Data Changed__ogtk.vi"("DBL"=w533) -> ("Changed"=w548:bool)
        n240 = case shown="True" w548 {
          tunnel: w533 -> [_ w649]
          frame False {
          }
          frame True {
            n241 = property on="Frequency" class="DigNum (strict)"("Val(Sgnl)"=w649) -> ()  [unwired: 2 in, 2 out]
          }
        }
        n242 = Bundle By Name(cluster=w557, "Desired Amplitude (V)"="Desired Amplitude (V)", "Width (ms) : 0.1"="Width (ms) : 0.1", "Frequency"=w533, "Needle Voltage"="Needle Voltage") -> (→"output cluster":T1)
        n243 = Build Array("Needle Voltage", "Desired Amplitude (V)", "Width (ms) : 0.1", w533) -> (w542:dbl[])
        n244 = Greater?(x=w542, y=dbl[] [0.0, 0.0, 0.0, 0.0]) -> (0:w540:bool[])
        n245 = And Array Elements(Boolean array=w540) -> (logical AND=w519:bool)
        "On/Off" <- w519
        n246 = event shown="[5] \"Width (ms) : 0.1\": Value Change" {
          selector: _ -> [_ _ _ _ _ _]
          dyn-events: _ -> [_ _ _ _ _ _]
          timeout: 100 -> [_ _ _ _ _ _]
          tunnel: w568 -> [w659 w701 w765 w849 w908 w967]
          tunnel: w570 -> [w674 w696 w764 w834 w893 w952]
          tunnel: w533 -> [w654 w710 w766 w851 w910 w969]
          tunnel: "Width (ms) : 0.1" -> [w655 w711 w767 w852 w911 w970]
          tunnel: [w673 w695 w752 w832 w891 w950] -> w539
          tunnel: w563 -> [w672 w709 w759 w850 w909 w968]
          tunnel: "Desired Amplitude (V)" -> [w657 w693 w748 _ w890 w949]
          tunnel: w555 -> [w663 w706 w762 w846 w905 w964]
          tunnel: w567 -> [w662 w705 w763 w845 w904 w963]
          tunnel: [w666 w708 w760 w848 w907 w966] -> w565
          tunnel: [FALSE ("y") FALSE ("y") TRUE ("y") FALSE ("y") FALSE ("y") FALSE ("y")] -> w536
          tunnel: w559 -> [w661 _ w754 w842 w901 w960]
          tunnel: w528 -> [w653 w692 _ w830 w888 w947]
          tunnel: w527 -> [w652 w691 _ w831 w887 w946]
          tunnel: w526 -> [w651 w690 _ w829 w886 w948]
          tunnel: w525 -> [w650 w689 _ w828 w889 w945]
          tunnel: [w653 w683 w747 w830 w888 w947] -> w524
          tunnel: [w652 w691 w747 w822 w887 w946] -> w523
          tunnel: [w651 w690 w747 w829 w886 w939] -> w522
          tunnel: [w650 w689 w747 w828 w878 w945] -> w521
          event Timeout {
            w656 = FALSE ("Blinking")
            n247 = event-data() -> ()  [unwired: 1 in, 2 out]
            n248 = local write "Actual Needle Output (V)"(w661) -> ()
            n249 = local write "Actual output Amplitude (V)"(w657) -> ()
            n250 = call "Gen_Square_0to10V.vi"("sampling info"=w659, "error in (no error)"=w674, "Width (ms)"=w655, "amplitude"=w657, "frequency"=w654) -> ("error out"=w669:errorcluster, "signal out"=w658:waveform(dbl))  [unwired: 5 in]
            n251 = Initialize Array(w661, w663) -> (w664:dbl[])
            n252 = local write "Actual output width (ms)"(w655) -> ()
            n253 = local write "Actual output Frequency"(w654) -> ()
            n254 = local write "Output waveform"(w658) -> ()
            n255 = Bundle By Name("Y"=w664, "dt"=w662) -> (w660:waveform(dbl))  [unwired: 1 in]
            n256 = Merge Signals(w658, w660) -> (w667:dynamicdata)
            n257 = call-poly <vilib>:"DAQmx Write.vi"("task/channels in"=w672, "data"=w667, "error in"=w669) -> ("task out"=w671:refnum<k21>, "error out"=w668:errorcluster)  [unwired: 10 in, 1 out]
            n258 = First Call?() -> (First Call?: T/F=w670:bool)
            n259 = case shown="True" w670 {
              tunnel: [w675 w680] -> w673
              tunnel: [w676 w679] -> w666
              tunnel: w671 -> [w676 w678]
              tunnel: w668 -> [w675 w677]
              frame False {
              }
              frame True {
                n260 = call <vilib>:"DAQmx Start Task.vi"("task/channels in"=w678, "error in"=w677) -> ("task out"=w679:refnum<k21>, "error out"=w680:errorcluster)  [unwired: 12 in]
              }
            }
            n261 = property on="Actual output Amplitude (V)" class="DigNum (strict)"("Blinking"=w656) -> ()  [unwired: 2 in, 2 out]
            n262 = property on="Actual Needle Output (V)" class="DigNum (strict)"("Blinking"=w656) -> ()  [unwired: 2 in, 2 out]
            n263 = property on="Actual output width (ms)" class="DigNum (strict)"("Blinking"=w656) -> ()  [unwired: 2 in, 2 out]
            n264 = property on="Actual output Frequency" class="DigNum (strict)"("Blinking"=w656) -> ()  [unwired: 2 in, 2 out]
          }
          event "Needle Voltage": Value Change {
            (unwired) "needle" ("name (unnamed)")
            w702 = 0.05 ("y")
            n265 = event-data() -> ("NewVal"=w682:dbl)  [unwired: 1 in, 4 out]
            n266 = Greater?(x=w682, y=w692) -> (0:w704:bool)
            n267 = Subtract(x=w682, y=w692) -> (x-y=w698:dbl)
            n268 = Subtract(x=w692, y=w682) -> (x-y=w699:dbl)
            n269 = Greater?(x=w698, y=w699) -> (0:w700:bool)
            n270 = Select(t=w698, s=w700, f=w699) -> (s? t:f=w697:dbl)
            n271 = Divide(x=w697, y=w702) -> (x/y=w703:dbl)
            n272 = To Long Integer(number=w703) -> (32bit integer=w681:i32)
            n273 = for {
              N: w681 -> [_]
              tunnel: w702 -> [w742]
              tunnel: w692 -> [w741]
              tunnel: w705 -> [w739]
              tunnel: w706 -> [w738]
              tunnel: [w721] -> w694
              tunnel: w711 -> [w719]
              tunnel: w693 -> [w720]
              tunnel: w710 -> [w734]
              tunnel: w696 -> [w733]
              shift-right: [w737] -> w708
              shift-left: w709 -> [w732]
              tunnel: w704 -> [w726]
              tunnel: w701 -> [w725]
              tunnel: [w715] -> w684
              tunnel: [w713] -> w685
              i -> [w743]
              stop <- w713 stop-if-true
              n274 = local write "Actual output Amplitude (V)"(w720) -> ()
              n275 = call "Gen_Square_0to10V.vi"("sampling info"=w725, "error in (no error)"=w733, "Width (ms)"=w719, "amplitude"=w720, "frequency"=w734) -> ("error out"=w735:errorcluster, "signal out"=w722:waveform(dbl))  [unwired: 5 in]
              n276 = Increment(x=w743) -> (x+1=w744:i32)
              n277 = property on="Actual Needle Output (V)" class="DigNum (strict)"("Blinking"=TRUE) -> ()  [unwired: 2 in, 2 out]
              n278 = local write "Output waveform"(w722) -> ()
              n279 = Multiply(x=w742, y=w744) -> (x*y=w728:dbl)
              n280 = Negate(x=w728) -> (-x=w729:dbl)
              n281 = Select(t=w728, s=w726, f=w729) -> (s? t:f=w727:dbl)
              n282 = Add(x=w741, y=w727) -> (x+y=w724:dbl)
              n283 = Divide(x=w724, y=1.0) -> (x/y=w717:dbl)
              n284 = Less Than 0?(x=w717) -> (x < 0?=w718:bool)
              n285 = Select(t=0.0, s=w718, f=w717) -> (s? t:f=w715:dbl)
              n286 = local write "Actual Needle Output (V)"(w715) -> ()
              n287 = Initialize Array(w715, w738) -> (w740:dbl[])
              n288 = Bundle By Name("Y"=w740, "dt"=w739) -> (w730:waveform(dbl))  [unwired: 1 in]
              n289 = Merge Signals(w722, w730) -> (w736:dynamicdata)
              n290 = local read "Abort Change"() -> (w714:bool)
              n291 = local read "stop"() -> (w712:bool)
              n292 = call-poly <vilib>:"DAQmx Write.vi"("task/channels in"=w732, "data"=w736, "error in"=w735) -> ("task out"=w737:refnum<k21>, "error out"=w721:errorcluster)  [unwired: 10 in, 1 out]
              n293 = Or(x=w714, y=w712) -> (x .or. y?=w713:bool)
              n294 = case shown="True" w713 {
                tunnel: w715 -> [_ w745]
                frame False {
                }
                frame True {
                  n295 = local write "Needle Voltage"(w745) -> ()
                }
              }
            }
            n296 = Equal To 0?(x=w681) -> (x = 0?=w687:bool)
            n297 = Not(x=w685) -> (.not. x?=w688:bool)
            n298 = Merge Errors(w694) -> (w695:errorcluster)
            n299 = Or(x=w688, y=w687) -> (x .or. y?=w686:bool)
            n300 = Select(t=w682, s=w686, f=w684) -> (s? t:f=w683:dbl)
          }
          event "stop": Value Change {
            w747 = 0.0 ("Width (ms) : 3.5")
            w751 = TRUE ("Blinking")
            n301 = event-data() -> ()  [unwired: 1 in, 1 out]
            n302 = property on="Actual Needle Output (V)" class="DigNum (strict)"("Blinking"=w751) -> ()  [unwired: 2 in, 2 out]
            n303 = property on="Actual output Amplitude (V)" class="DigNum (strict)"("Blinking"=w751) -> ()  [unwired: 2 in, 2 out]
            n304 = Multiply(x=w754, y=20.0 ("x")) -> (x*y=w756:dbl)
            n305 = Multiply(x=20.0, y=w748) -> (x*y=w746:dbl)
            n306 = Greater?(x=w756, y=w746) -> (0:w755:bool)
            n307 = Select(t=w756, s=w755, f=w746) -> (s? t:f=w749:dbl)
            n308 = Increment(x=w749) -> (x+1=w750:dbl)
            n309 = for {
              N: w750 -> [w775]
              tunnel: w767 -> [w788]
              tunnel: w766 -> [w787]
              tunnel: w765 -> [w781]
              tunnel: w748 -> [w789]
              tunnel: w762 -> [w779]
              tunnel: w763 -> [w778]
              tunnel: [w778] -> _ mode=indexing
              shift-right: [w783] -> w753
              shift-left: w764 -> [w782]
              tunnel: w754 -> [w771]
              tunnel: w759 -> [w785]
              tunnel: [w786] -> w760
              i -> [w777]
              n310 = Subtract(x=w775, y=1) -> (x-y=w774:i32)
              n311 = Wait (ms)(milliseconds to wait=u32 250) -> ()  [unwired: 1 out]
              n312 = Equal?(x=w774, y=w777) -> (x = y?=w776:bool)
              n313 = case shown="True" w776 {
                tunnel: w789 -> [w812 _]
                tunnel: w788 -> [w811 _]
                tunnel: w787 -> [w810 _]
                tunnel: [w809 w818] -> w784
                tunnel: w782 -> [w808 w818]
                tunnel: w781 -> [w804 _]
                tunnel: [w803 w819] -> w780
                tunnel: w775 -> [w800 _]
                tunnel: w779 -> [w796 w814]
                tunnel: w778 -> [w798 w816]
                tunnel: w777 -> [w790 _]
                tunnel: w771 -> [w799 _]
                tunnel: [w792 w817] -> w770
                frame False {
                  n314 = Divide(x=w799, y=w800) -> (x/y=w802:dbl)
                  n315 = Divide(x=w812, y=w800) -> (x/y=w807:dbl)
                  n316 = Multiply(x=w802, y=w790) -> (x*y=w801:dbl)
                  n317 = Multiply(x=w807, y=w790) -> (x*y=w806:dbl)
                  n318 = Subtract(x=w799, y=w801) -> (x-y=w793:dbl)
                  n319 = Subtract(x=w812, y=w806) -> (x-y=w805:dbl)
                  n320 = local write "Actual output Amplitude (V)"(w805) -> ()
                  n321 = call "Gen_Square_0to10V.vi"("sampling info"=w804, "error in (no error)"=w808, "Width (ms)"=w811, "amplitude"=w805, "frequency"=w810) -> ("error out"=w809:errorcluster, "signal out"=w792:waveform(dbl))  [unwired: 5 in]
                  n322 = Divide(x=w793, y=1.0) -> (x/y=w794:dbl)
                  n323 = local write "Actual Needle Output (V)"(w794) -> ()
                  n324 = Initialize Array(w794, w796) -> (w797:dbl[])
                  n325 = Bundle By Name("Y"=w797, "dt"=w798) -> (w791:waveform(dbl))  [unwired: 1 in]
                  n326 = Merge Signals(w792, w791) -> (w803:dynamicdata)
                }
                frame True {
                  w815 = 0.0 ("element")
                  n327 = local write "Actual Needle Output (V)"(w815) -> ()
                  n328 = local write "Needle Voltage"(w815) -> ()
                  n329 = local write "Desired Amplitude (V)"(w815) -> ()
                  n330 = local write "Actual output Amplitude (V)"(w815) -> ()
                  n331 = Initialize Array(w815, w814) -> (w813:dbl[])
                  n332 = Bundle By Name("Y"=w813, "dt"=w816) -> (w817:waveform(dbl))  [unwired: 1 in]
                  n333 = Merge Signals(w817, w817) -> (w819:dynamicdata)
                }
              }
              n334 = local write "Output waveform"(w770) -> ()
              n335 = call-poly <vilib>:"DAQmx Write.vi"("task/channels in"=w785, "data"=w780, "error in"=w784) -> ("task out"=w786:refnum<k21>, "error out"=w783:errorcluster)  [unwired: 10 in, 1 out]
            }
            n336 = flat-sequence {
              tunnel: w753 -> [w769]
              tunnel: [w769] -> w752
              frame #0 {
                w768 = TRUE ("Finished")
                n337 = local write "stop"(w768) -> ()
                "Finished" <- w768
              }
            }
          }
          event "Desired Amplitude (V)": Value Change {
            w839 = 0.05 ("y")
            n338 = event-data() -> ("NewVal"=w821:dbl)  [unwired: 1 in, 1 out]
            n339 = local write "Actual Needle Output (V)"(w842) -> ()
            n340 = Greater?(x=w821, y=w831) -> (0:w841:bool)
            n341 = Subtract(x=w821, y=w831) -> (x-y=w837:dbl)
            n342 = Subtract(x=w831, y=w821) -> (x-y=w835:dbl)
            n343 = Initialize Array(w842, w846) -> (w844:dbl[])
            n344 = Greater?(x=w837, y=w835) -> (0:w838:bool)
            n345 = Bundle By Name("Y"=w844, "dt"=w845) -> (w843:waveform(dbl))  [unwired: 1 in]
            n346 = Select(t=w837, s=w838, f=w835) -> (s? t:f=w836:dbl)
            n347 = Quotient & Remainder(x=w836, y=w839) -> (floor(x/y)=w840:dbl)  [unwired: 1 out]
            n348 = To Long Integer(number=w840) -> (32bit integer=w820:i32)
            n349 = for {
              N: w820 -> [_]
              tunnel: w852 -> [w875]
              tunnel: w851 -> [w874]
              tunnel: w831 -> [w872]
              tunnel: w834 -> [w871]
              tunnel: [w869] -> w833
              tunnel: w849 -> [w867]
              tunnel: w839 -> [w864]
              tunnel: w843 -> [w862]
              shift-right: [w868] -> w848
              shift-left: w850 -> [w870]
              tunnel: w841 -> [w858]
              tunnel: [w856] -> w823
              tunnel: [w854] -> w824
              i -> [w873]
              stop <- w854 stop-if-true
              n350 = Increment(x=w873) -> (x+1=w866:i32)
              n351 = property on="Actual output Amplitude (V)" class="DigNum (strict)"("Blinking"=TRUE) -> ()  [unwired: 2 in, 2 out]
              n352 = Multiply(x=w864, y=w866) -> (x*y=w859:dbl)
              n353 = Negate(x=w859) -> (-x=w861:dbl)
              n354 = Select(t=w859, s=w858, f=w861) -> (s? t:f=w860:dbl)
              n355 = Add(x=w872, y=w860) -> (x+y=w856:dbl)
              n356 = local write "Actual output Amplitude (V)"(w856) -> ()
              n357 = call "Gen_Square_0to10V.vi"("sampling info"=w867, "error in (no error)"=w871, "Width (ms)"=w875, "amplitude"=w856, "frequency"=w874) -> ("error out"=w876:errorcluster, "signal out"=w857:waveform(dbl))  [unwired: 5 in]
              n358 = local write "Output waveform"(w857) -> ()
              n359 = Merge Signals(w857, w862) -> (w863:dynamicdata)
              n360 = call-poly <vilib>:"DAQmx Write.vi"("task/channels in"=w870, "data"=w863, "error in"=w876) -> ("task out"=w868:refnum<k21>, "error out"=w869:errorcluster)  [unwired: 10 in, 1 out]
              n361 = local read "Abort Change"() -> (w855:bool)
              n362 = local read "stop"() -> (w853:bool)
              n363 = Or(x=w855, y=w853) -> (x .or. y?=w854:bool)
              n364 = case shown="True" w854 {
                tunnel: w856 -> [_ w877]
                frame False {
                }
                frame True {
                  n365 = local write "Desired Amplitude (V)"(w877) -> ()
                }
              }
            }
            n366 = Equal To 0?(x=w820) -> (x = 0?=w826:bool)
            n367 = Not(x=w824) -> (.not. x?=w827:bool)
            n368 = Merge Errors(w833) -> (w832:errorcluster)
            n369 = Or(x=w827, y=w826) -> (x .or. y?=w825:bool)
            n370 = Select(t=w821, s=w825, f=w823) -> (s? t:f=w822:dbl)
          }
          event "Frequency": Value Change {
            w898 = 0.5 ("y")
            n371 = event-data() -> ("NewVal"=w880:dbl)  [unwired: 1 in, 1 out]
            n372 = local write "Actual Needle Output (V)"(w901) -> ()
            n373 = Greater?(x=w880, y=w889) -> (0:w900:bool)
            n374 = Subtract(x=w880, y=w889) -> (x-y=w896:dbl)
            n375 = Subtract(x=w889, y=w880) -> (x-y=w894:dbl)
            n376 = Initialize Array(w901, w905) -> (w903:dbl[])
            n377 = Greater?(x=w896, y=w894) -> (0:w897:bool)
            n378 = Bundle By Name("Y"=w903, "dt"=w904) -> (w902:waveform(dbl))  [unwired: 1 in]
            n379 = Select(t=w896, s=w897, f=w894) -> (s? t:f=w895:dbl)
            n380 = Quotient & Remainder(x=w895, y=w898) -> (floor(x/y)=w899:dbl)  [unwired: 1 out]
            n381 = To Long Integer(number=w899) -> (32bit integer=w879:i32)
            n382 = for {
              N: w879 -> [_]
              tunnel: w911 -> [w934]
              tunnel: w910 -> [_]
              tunnel: w889 -> [w932]
              tunnel: w893 -> [w931]
              tunnel: [w929] -> w892
              tunnel: w908 -> [w927]
              tunnel: w898 -> [w925]
              tunnel: w902 -> [w923]
              shift-right: [w928] -> w907
              shift-left: w909 -> [w930]
              tunnel: w900 -> [w919]
              tunnel: w890 -> [w916]
              tunnel: [w915] -> w881
              tunnel: [w913] -> w882
              i -> [w933]
              stop <- w913 stop-if-true
              n383 = Increment(x=w933) -> (x+1=w926:i32)
              n384 = Multiply(x=w925, y=w926) -> (x*y=w920:dbl)
              n385 = property on="Actual output Frequency" class="DigNum (strict)"("Blinking"=TRUE) -> ()  [unwired: 2 in, 2 out]
              n386 = Negate(x=w920) -> (-x=w922:dbl)
              n387 = Select(t=w920, s=w919, f=w922) -> (s? t:f=w921:dbl)
              n388 = Add(x=w932, y=w921) -> (x+y=w915:dbl)
              n389 = call "Gen_Square_0to10V.vi"("sampling info"=w927, "error in (no error)"=w931, "Width (ms)"=w934, "amplitude"=w916, "frequency"=w915) -> ("error out"=w935:errorcluster, "signal out"=w918:waveform(dbl))  [unwired: 5 in]
              n390 = local write "Actual output Frequency"(w915) -> ()
              n391 = local write "Output waveform"(w918) -> ()
              n392 = Merge Signals(w918, w923) -> (w924:dynamicdata)
              n393 = local read "Abort Change"() -> (w914:bool)
              n394 = call-poly <vilib>:"DAQmx Write.vi"("task/channels in"=w930, "data"=w924, "error in"=w935) -> ("task out"=w928:refnum<k21>, "error out"=w929:errorcluster)  [unwired: 10 in, 1 out]
              n395 = local read "stop"() -> (w912:bool)
              n396 = Or(x=w914, y=w912) -> (x .or. y?=w913:bool)
              n397 = case shown="True" w913 {
                tunnel: w915 -> [_ w936]
                frame False {
                }
                frame True {
                  n398 = local write "Frequency"(w936) -> ()
                }
              }
            }
            n399 = Equal To 0?(x=w879) -> (x = 0?=w884:bool)
            n400 = Not(x=w882) -> (.not. x?=w885:bool)
            n401 = Merge Errors(w892) -> (w891:errorcluster)
            n402 = Or(x=w885, y=w884) -> (x .or. y?=w883:bool)
            n403 = Select(t=w880, s=w883, f=w881) -> (s? t:f=w878:dbl)
          }
          event "Width (ms) : 0.1": Value Change {
            w957 = 0.1 ("y")
            n404 = event-data() -> ("NewVal"=w937:dbl)  [unwired: 1 in, 1 out]
            n405 = local write "Actual Needle Output (V)"(w960) -> ()
            n406 = Greater?(x=w937, y=w948) -> (0:w959:bool)
            n407 = Subtract(x=w937, y=w948) -> (x-y=w955:dbl)
            n408 = Subtract(x=w948, y=w937) -> (x-y=w953:dbl)
            n409 = Initialize Array(w960, w964) -> (w962:dbl[])
            n410 = Greater?(x=w955, y=w953) -> (0:w956:bool)
            n411 = Bundle By Name("Y"=w962, "dt"=w963) -> (w961:waveform(dbl))  [unwired: 1 in]
            n412 = Select(t=w955, s=w956, f=w953) -> (s? t:f=w954:dbl)
            n413 = Quotient & Remainder(x=w954, y=w957) -> (floor(x/y)=w958:dbl)  [unwired: 1 out]
            n414 = To Long Integer(number=w958) -> (32bit integer=w941:i32)
            n415 = for {
              N: w941 -> [_]
              tunnel: w970 -> [_]
              tunnel: w969 -> [w993]
              tunnel: w948 -> [w991]
              tunnel: w952 -> [w990]
              tunnel: [w988] -> w951
              tunnel: w967 -> [w986]
              tunnel: w957 -> [w984]
              tunnel: w961 -> [w982]
              shift-right: [w987] -> w966
              shift-left: w968 -> [w989]
              tunnel: w959 -> [w978]
              tunnel: w949 -> [w976]
              tunnel: [w974] -> w938
              tunnel: [w972] -> w944
              i -> [w992]
              stop <- w972 stop-if-true
              n416 = Increment(x=w992) -> (x+1=w985:i32)
              n417 = Multiply(x=w984, y=w985) -> (x*y=w979:dbl)
              n418 = property on="Actual output width (ms)" class="DigNum (strict)"("Blinking"=TRUE) -> ()  [unwired: 2 in, 2 out]
              n419 = Negate(x=w979) -> (-x=w981:dbl)
              n420 = Select(t=w979, s=w978, f=w981) -> (s? t:f=w980:dbl)
              n421 = Add(x=w991, y=w980) -> (x+y=w974:dbl)
              n422 = call "Gen_Square_0to10V.vi"("sampling info"=w986, "error in (no error)"=w990, "Width (ms)"=w974, "amplitude"=w976, "frequency"=w993) -> ("error out"=w994:errorcluster, "signal out"=w977:waveform(dbl))  [unwired: 5 in]
              n423 = local write "Actual output width (ms)"(w974) -> ()
              n424 = local write "Output waveform"(w977) -> ()
              n425 = Merge Signals(w977, w982) -> (w983:dynamicdata)
              n426 = local read "Abort Change"() -> (w973:bool)
              n427 = call-poly <vilib>:"DAQmx Write.vi"("task/channels in"=w989, "data"=w983, "error in"=w994) -> ("task out"=w987:refnum<k21>, "error out"=w988:errorcluster)  [unwired: 10 in, 1 out]
              n428 = local read "stop"() -> (w971:bool)
              n429 = Or(x=w971, y=w973) -> (x .or. y?=w972:bool)
              n430 = case shown="True" w972 {
                tunnel: w974 -> [_ w995]
                frame False {
                }
                frame True {
                  n431 = local write "Width (ms) : 0.1"(w995) -> ()
                }
              }
            }
            n432 = Equal To 0?(x=w941) -> (x = 0?=w942:bool)
            n433 = Not(x=w944) -> (.not. x?=w943:bool)
            n434 = Or(x=w943, y=w942) -> (x .or. y?=w940:bool)
            n435 = Merge Errors(w951) -> (w950:errorcluster)
            n436 = Select(t=w937, s=w940, f=w938) -> (s? t:f=w939:dbl)
          }
        }
        n437 = call-poly <userlib>:"Data Changed__ogtk.vi"("Boolean"=w519) -> ("Changed"=w520:bool)
        n438 = And(x=w536, y=w519) -> (x .and. y?=w535:bool)
        n439 = Or(x=w535, y=w520) -> (x .or. y?=w537:bool)
        n440 = local read "Testing"() -> (w515:bool)
        n441 = case shown="True" w537 {
          tunnel: w519 -> [_ w580]
          tunnel: w539 -> [w577 w585]
          tunnel: [w577 w584] -> w538
          tunnel: w535 -> [_ w579]
          tunnel: w518 -> [w576 w583]
          tunnel: [w576 w582] -> w517
          frame False {
          }
          frame True {
            n442 = Select(t=FALSE, s=w579, f=w580) -> (s? t:f=w581:bool)
            n443 = case shown="False" w581 {
              tunnel: w585 -> [w607 w648]
              tunnel: [w604 w648] -> w584
              tunnel: w583 -> [w586 _]
              tunnel: [w586 w646] -> w582
              frame False {
                n444 = Get Date/Time In Seconds() -> (seconds since 1Jan1904=w610:timestamp)
                n445 = call "LV_to_int_time.vi"("error in (no error)"=w607, "Time Stamp"=w610) -> ("error out"=w608:errorcluster, "Integer Time"=w587:i64)  [unwired: 7 in]
                n446 = call "connect in.vi"("error in (no error)"=w608) -> ("error out"=w602:errorcluster, "Database Connection"=w603:T4)  [unwired: 7 in]
                n447 = call-poly <vilib>:"DB Tools Execute Query.vi"("error in (no error)"=w602, "SQL query"="SELECT id_experiment_settings\nFROM experiment_settings_small\nORDER BY integer_timestamp DESC\nLIMIT 1; ", "connection reference"=w603) -> ("error out"=w600:errorcluster, "recordset reference"=w601:T5)  [unwired: 5 in]
                n448 = call-poly <vilib>:"DB Tools Fetch Recordset Data.vi"("error in (no error)"=w600, "recordset reference"=w601) -> ("error out"=w589:errorcluster, "recordset data"=w595:variant[][], "recordset reference out"=w599:T5)  [unwired: 3 in]
                n449 = Index Array(array=w595, index (row)=0, index (col)=0 ("disabled index (col)")) -> (element=w592:variant)
                n450 = xnode "Database Variant To Data"("database variant"=w592, "error in (no error)"=w589, "type"=0) -> ("data"=w590:i32, "error out"=w588:errorcluster)
                n451 = call-poly <vilib>:"DB Tools Free Object.vi"("error in (no error)"=w588, "recordset reference"=w599) -> ("error out"=w597:errorcluster, "connection reference"=w598:T4)  [unwired: 8 in]
                n452 = Bundle("Integer Time"=w586, "Integer Time"=w587, "data"=w590) -> (w609:T9)  [unwired: 1 in]
                n453 = call <vilib>:"DB Tools Insert Data.vi"("create table? (F)"=FALSE, "data"=w609, "error in (no error)"=w597, "table"="run_times_small", "connection reference"=w598) -> ("error out"=w605:errorcluster, "connection reference out"=w612:T4)  [unwired: 5 in]
                n454 = call "connect out.vi"("error in (no error)"=w602, "connection reference"=w612) -> ("error out"=w606:errorcluster)  [unwired: 9 in]
                n455 = Merge Errors(w605, w606) -> (w604:errorcluster)
              }
              frame True {
                n456 = Get Date/Time In Seconds() -> (seconds since 1Jan1904=w647:timestamp)
                n457 = call "LV_to_int_time.vi"("Time Stamp"=w647) -> ("Integer Time"=w646:i64)  [unwired: 8 in, 1 out]
              }
            }
          }
        }
        n458 = Unbundle By Name(w538) -> ("status"=w514:bool)
        n459 = call <vilib>:"Simple Error Handler.vi"("type of dialog (OK msg:1)"=w561, "error in (no error)"=w538) -> ("error?"=w516:bool, "error out"=w562:errorcluster)  [unwired: 3 in, 3 out]
        n460 = Not(x=w515) -> (.not. x?=w509:bool)
        n461 = case shown="False" w515 {
          tunnel: w516 -> [w571 w572]
          tunnel: [w571 w572] -> w512
          frame False {
            n462 = property on="error?" class="Bool (strict)"("Val(Sgnl)"=w571) -> ()  [unwired: 2 in, 2 out]
          }
          frame True {
          }
        }
        n463 = And(x=w509, y=w514) -> (x .and. y?=w513:bool)
        n464 = Or(x=w513, y=w536) -> (x .or. y?=w511:bool)
        n465 = And(x=w509, y=w512) -> (x .and. y?=→"error?":bool)
        "Execution Number:" <- w569
      }
      n466 = call <vilib>:"DAQmx Clear Task.vi"("task in"=w61, "error in"=w76) -> ("error out"=w75:errorcluster)  [unwired: 13 in]
      n467 = call <vilib>:"DAQmx Stop Task.vi"("task/channels in"=w98, "error in"=w97) -> ("task out"=w94:refnum<k21>, "error out"=w93:errorcluster)  [unwired: 12 in]
      n468 = call <vilib>:"DAQmx Stop Task.vi"("task/channels in"=w96, "error in"=w95) -> ("task out"=w92:refnum<k21>, "error out"=w91:errorcluster)  [unwired: 12 in]
      n469 = call <vilib>:"DAQmx Clear Task.vi"("task in"=w94, "error in"=w93) -> ("error out"=w86:errorcluster)  [unwired: 13 in]
      n470 = call <vilib>:"DAQmx Clear Task.vi"("task in"=w92, "error in"=w91) -> ("error out"=w85:errorcluster)  [unwired: 13 in]
      n471 = Merge Errors(w86, w85, w57) -> (w83:errorcluster)
      n472 = call <vilib>:"DAQmx Clear Task.vi"("task in"=w112, "error in"=w108) -> ("error out"=w111:errorcluster)  [unwired: 13 in]
      n473 = call <vilib>:"Simple Error Handler.vi"("type of dialog (OK msg:1)"=w123, "error in (no error)"=w111) -> ("error out"=w110:errorcluster)  [unwired: 3 in, 4 out]
      n474 = Merge Errors(w110, w83, w75, w84) -> (w106:errorcluster)
      n475 = while {
        tunnel: [w290] -> w105
        tunnel: w106 -> [w290]
        stop <- w291 stop-if-true
        # "Loop to ask if the batteries are off"
        n476 = Two Button Dialog(message="Have you turned off the High voltage?", 1:"No, thank you for reminding me! I'll go do that right now!" ("button name (\"OK\")"), 2:"Yes, of course I have." ("T button name (\"OK\")")) -> (T button?=w291:bool)
      }
    }
    frame Error {
    }
  }
  "error out" <- w50
